vi "I2C Open.vi"(7 "I2C Channel (0)":u8, 8 "Error In":errorcluster, 11 "LINX Resource":T1) -> (0 "Error Out":errorcluster, 3 "LINX Resource":T1)   [LabVIEW 2014, in "LMH-LINX.lvlib"]
doc: "Open the specified I2C channel. If the LINX device has a single I2C master it is channel 0. If the LINX device has more than one I2C master the logical first I2C master is channel 0, the next is channel 1, etc.\n\nFor example on myRIO:\nA/I2C maps to LINX I2C Channel 0\nB/I2C maps to LINX I2C Channel 1"
uses:
  LMH-LINX.lvlib
  Private/Type Defs/LINX Ref.ctl
  Private/Type Defs/Platform.ctl
  Private/Type Defs/Interface.ctl
  Private/Device/Type Defs/LINX Device Config.ctl
  Private/Device/Type Defs/TCP Config.ctl
  Private/Device/Type Defs/Channels.ctl
  Private/Type Defs/Peripheral.ctl
  Private/Type Defs/Channel FGV States.ctl
  Private/Device/Device.lvlib
  Private/myRIO/myRIO.lvlib
  <vilib>/myRIO/Instrument Drivers/Onboard IO/I2C/I2C.lvlib
  <vilib>/myRIO/Instrument Drivers/Onboard IO/I2C/typedefs/I2C Transfer Rate.ctl
  <vilib>/myRIO/Instrument Drivers/Onboard IO/I2C/typedefs/I2C User Configuration.ctl
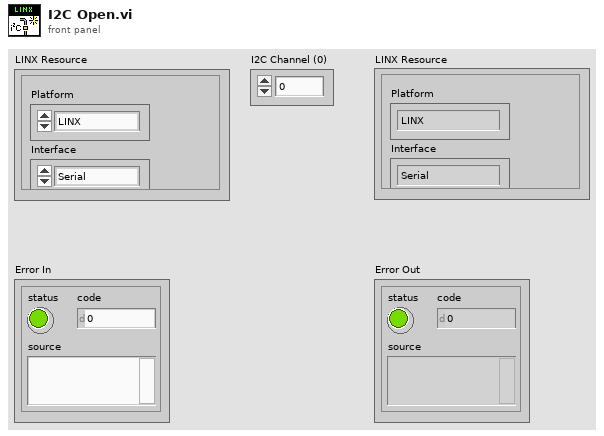
[diagram p1: front panel]
types:
  T1 = typedef "LMH-LINX.lvlib/LINX Ref.ctl" = cluster{"Platform":T2, "Interface":T3, "LINX Device Config":T4}
  T2 = typedef "LMH-LINX.lvlib/Platform.ctl" = enum16{"LINX", "myRIO"}
  T3 = typedef "LMH-LINX.lvlib/Interface.ctl" = enum16{"Serial", "TCP"}
  T4 = typedef "LMH-LINX.lvlib/Device.lvlib/LINX Device Config.ctl" = cluster{"Interface":T3, "COM Port":refnum<visa-resource-name>, "TCP Configuration":T5, "Device Family":u8, "Device ID":u8, "Device Name":string, "TCP Ref":refnum<k5>, "Channels":T6}
  T5 = typedef "LMH-LINX.lvlib/Device.lvlib/TCP Config.ctl" = cluster{"IP Address":string, "Port":u16}
  T6 = typedef "LMH-LINX.lvlib/Channels.ctl" = cluster{"DI":u8[], "DO":u8[], "AI":u8[], "AO":u8[], "PWM":u8[], "QE":u8[], "UART":u8[], "I2C 2":u8[], "SPI":u8[], "CAN":u8[], "Servo":u8[], "AI Ref (V)":dbl, "AO Ref (V)":dbl, "AO Resolution (Bits)":u8}
  T7 = typedef "LMH-LINX.lvlib/Peripheral.ctl" = enum8{"DI", "DO", "AI", "AO", "PWM", "QE", "UART", "I2C", "SPI", "CAN", "Servo"}
  T8 = typedef "LMH-LINX.lvlib/Channel FGV States.ctl" = enum16{"Initialize", "Get", "Set"}
  T9 = typedef "I2C.lvlib/I2C User Configuration.ctl" = cluster{"I2C Transfer Rate":T10}
  T10 = typedef "I2C.lvlib/I2C Transfer Rate.ctl" = enum16{"Standard mode (100 kbps)", "Fast mode (400 kbps)"}
  T11 = typedef "I2C.lvlib/I2C Reference.ctl" = cluster{"myRIO Reference":T12, "I2C Channels Enum":T16, "I2C Configuration":T17}
  T12 = typedef "myRIO Generic Hardware Reference.ctl" = cluster{"myRIO Model":T13, "myRIO Hardware Reference":T14}
  T13 = typedef "Hardware Version Enum.ctl" = enum16{"Unknown", "myRIO-1900", "myRIO-1950"}
  T14 = typedef "myRIO v1.0 Reference.ctl" = cluster{"Generic FPGA Reference":T15, "Allow multiple opens":bool}
  T15 = typedef "Generic FPGA Reference.ctl" = refnum<k20>
  T16 = typedef "I2C Channels Enum.ctl" = enum16{"Not Connected", "A/I2C", "B/I2C"}
  T17 = typedef "I2C.lvlib/I2C Configuration.ctl" = cluster{"I2C Transfer Rate":T10}
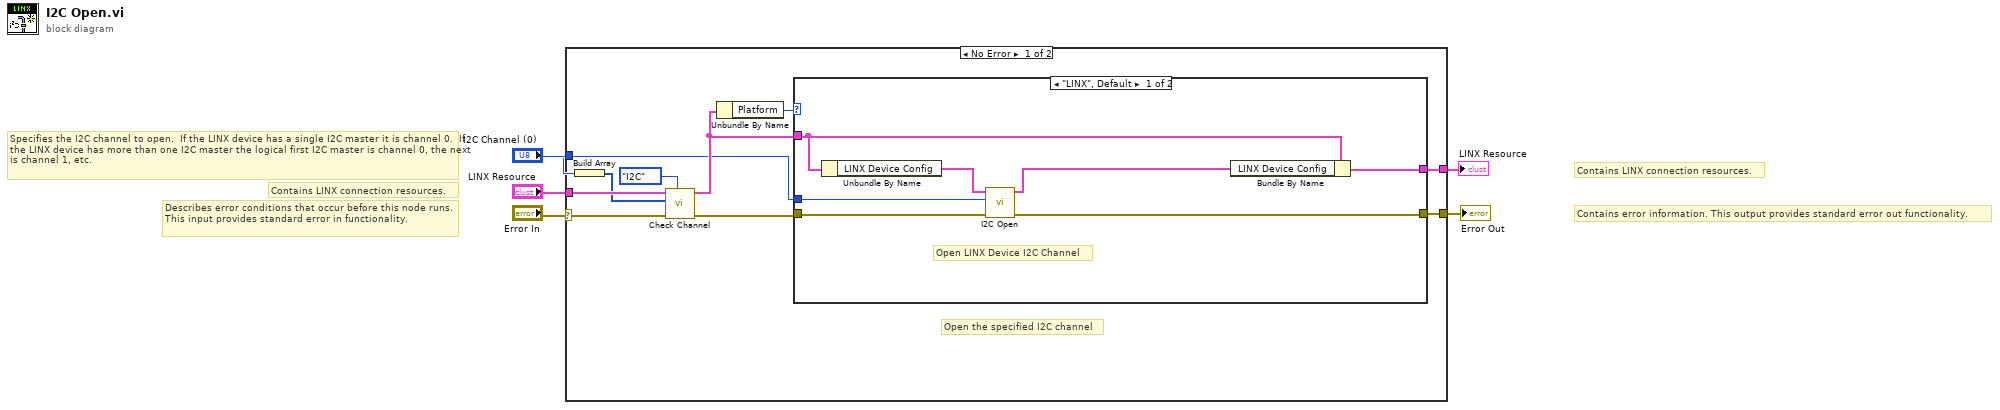
[diagram p0: block diagram]
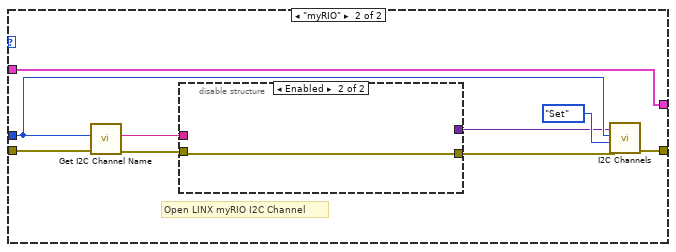
[diagram p2: hidden frame]
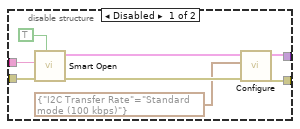
[diagram p3: hidden frame]
diagram:
  # "Specifies the I2C channel to open.  If the LINX device has a single I2C master it is channel 0.  If the LINX device has more than one I2C master the logical first I2C master is channel 0, the next is channel 1, etc."
  # "Contains LINX connection resources."
  # "Contains error information. This output provides standard error out functionality."
  # "Contains LINX connection resources."
  # "Describes error conditions that occur before this node runs. This input provides standard error in functionality."
  n1 = case shown="No Error" "Error In" {
    selector: "Error In" -> [w6 w42]
    tunnel: [w14 w42] -> w5
    tunnel: [w13 w41] -> w4
    tunnel: "LINX Resource" -> [w12 w41]
    tunnel: "I2C Channel (0)" -> [w8 _]
    frame No Error {
      # "Open the specified I2C channel"
      n2 = Build Array(w8) -> (w9:u8[])
      n3 = call "Check Channel.vi"("Peripheral"=Peripheral."I2C", "Error In"=w6, "Channels"=w9, "LINX Resource"=w12) -> ("Error Out"=w10:errorcluster, "LINX Resource"=w11:T1)  [unwired: 5 in, 1 out]
      n4 = Unbundle By Name(w11) -> ("Platform"=w15:T2)
      n5 = case shown="\"LINX\", Default" w15 {
        tunnel: w10 -> [w20 w27]
        tunnel: w11 -> [w22 w31]
        tunnel: [w19 w30] -> w14
        tunnel: [w21 w31] -> w13
        tunnel: w8 -> [w16 w28]
        frame "LINX", Default {
          # "Open LINX Device I2C Channel"
          n6 = Unbundle By Name(w22) -> ("LINX Device Config"=w17:T4)
          n7 = call "I2C Open.vi"("Error In"=w20, "I2C Channel (0)"=w16, "LINX Device Config"=w17) -> ("Error Out"=w19:errorcluster, "LINX Device Config"=w18:T4)  [unwired: 7 in]
          n8 = Bundle By Name(cluster=w22, "LINX Device Config"=w18) -> (w21:T1)
        }
        frame "myRIO" {
          # "Open LINX myRIO I2C Channel"
          n9 = call "Get I2C Channel Name.vi"("Error In"=w27, "I2C Channel"=w28) -> ("Error Out"=w25:errorcluster, "myRIO I2C Channels"=w24:string)  [unwired: 8 in]
          n10 = disable-structure shown="Enabled" {
            disable-tunnel: [w34 w40] -> w26
            disable-tunnel: w25 -> [w38 w40]
            disable-tunnel: w24 -> [w37 _]
            disable-tunnel: [w35 _] -> w23
            frame Disabled {
              n11 = call <vilib>:"Smart Open.vi"("Allow multiple opens?"=TRUE, "error in (no error)"=w38, "Channel Name"=w37) -> ("error out"=w33:errorcluster, "I2C Ref Out"=w36:T11)  [unwired: 7 in]
              n12 = call <vilib>:"Configure.vi"("error in (no error)"=w33, "I2C User Configuration"=T9 {"I2C Transfer Rate"=enum."Standard mode (100 kbps)"}, "I2C Ref In"=w36) -> ("error out"=w34:errorcluster, "I2C Ref Out"=w35:T11)  [unwired: 7 in]
            }
            frame Enabled {
            }
          }
          n13 = call "I2C Channels.vi"("Error In"=w26, "Channel State"=Channel_FGV_States."Set", "Channel Number"=w28, "I2C Channel"=w23) -> ("Error Out"=w30:errorcluster)  [unwired: 6 in, 1 out]
        }
      }
    }
    frame Error {
    }
  }
  "Error Out" <- w5
  "LINX Resource" <- w4
